vi "Get Rx Hardware Channel Data.vi"(8 "error in":errorcluster, 11 "custom device ref in":T1 format="%.0x") -> (0 "error out":errorcluster, 1 "Rx hardware channel data":T2[](array[typedef]) {"labels settings for RT"."Label Timestamp Channel Data Reference" format="%.0x"; "labels settings for RT"."Word Initial Raw Value" format="%032.0f"; "labels settings for RT"."Label Disable/Trigger Channel Reference" format="%.0x"; "labels settings for RT"."parameter driver data"."Tx parameter refs" format="%.0x"; "labels settings for RT"."parameter driver data"."Rx block data refs"."Data Reference" format="%.0x"; "labels settings for RT"."SDI" format="%02b"; "labels settings for RT"."label" format="%.0o"}, 2 "incoming channels":T1[](array[typedef]) format="%.0x", 3 "custom device ref out":T1 format="%.0x")   [LabVIEW 2020]
uses:
  <vilib>/NI VeriStand/Custom Device API/Custom Device API.lvlib
  Scripting/Ballard ARINC 429 Scripting.lvlib
  <vilib>/NI VeriStand/Custom Device API/Data Access Type.ctl
  <vilib>/NI VeriStand/Custom Device API/Custom Device Item Ref.ctl
  Label.ctl
  Encoding and Decoding/Encoding.ctl
  Encoding and Decoding/Encoding and Decoding.lvlib
  <vilib>/NI VeriStand/Custom Device API/Data Reference.ctl
  <vilib>/NI VeriStand/Custom Device API/Block Data Reference.ctl
  RT Parameters.ctl
  RT Label Settings.ctl
  RT Hardware Channel Settings.ctl
  Transfer Type.ctl
  Parameter Definition.ctl
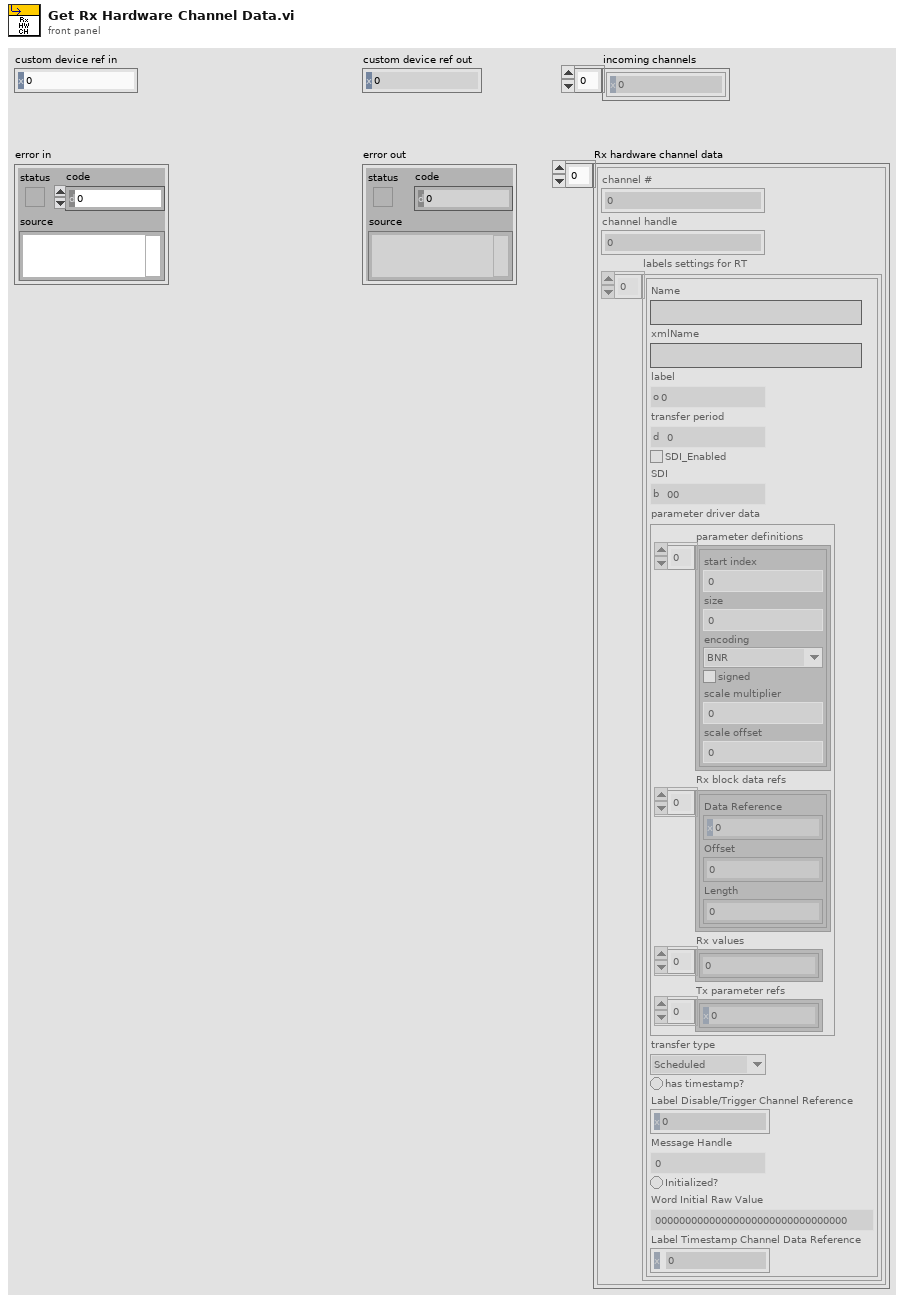
[diagram p1: front panel]
types:
  T1 = typedef "Custom Device API.lvlib/Custom Device Item Ref.ctl" = u64
  T2 = typedef "RT Hardware Channel Settings.ctl" = cluster{"channel #":u16, "channel handle":u64, "labels settings for RT":T3[]}
  T3 = typedef "RT Label Settings.ctl" = cluster{"Name":string, "xmlName":string, "label":T4, "transfer period":u32, "SDI_Enabled":bool, "SDI":u8, "parameter driver data":T5, "transfer type":T10, "has timestamp?":bool, "Label Disable/Trigger Channel Reference":T1, "Message Handle":u64, "Initialized?":bool, "Word Initial Raw Value":u32, "Label Timestamp Channel Data Reference":T9}
  T4 = typedef "Label.ctl" = u8
  T5 = typedef "RT Parameters.ctl" = cluster{"parameter definitions":T6[], "Rx block data refs":T8[], "Rx values":dbl[], "Tx parameter refs":T1[]}
  T6 = typedef "Parameter Definition.ctl" = cluster{"start index":i32, "size":i32, "encoding":T7, "signed":bool, "scale multiplier":dbl, "scale offset":dbl}
  T7 = typedef "Encoding and Decoding.lvlib/Encoding.ctl" = enum16{"BNR", "BCD", "Discrete"}
  T8 = typedef "Custom Device API.lvlib/Block Data Reference.ctl" = cluster{"Data Reference":T9, "Offset":u64, "Length":u64}
  T9 = typedef "Custom Device API.lvlib/Data Reference.ctl" = i32
  T10 = typedef "Transfer Type.ctl" = enum16{"Scheduled", "Acyclic", "Block", "Strobe"}
  T11 = typedef "Custom Device API.lvlib/Data Access Type.ctl" = enum16{"Read", "Write"}
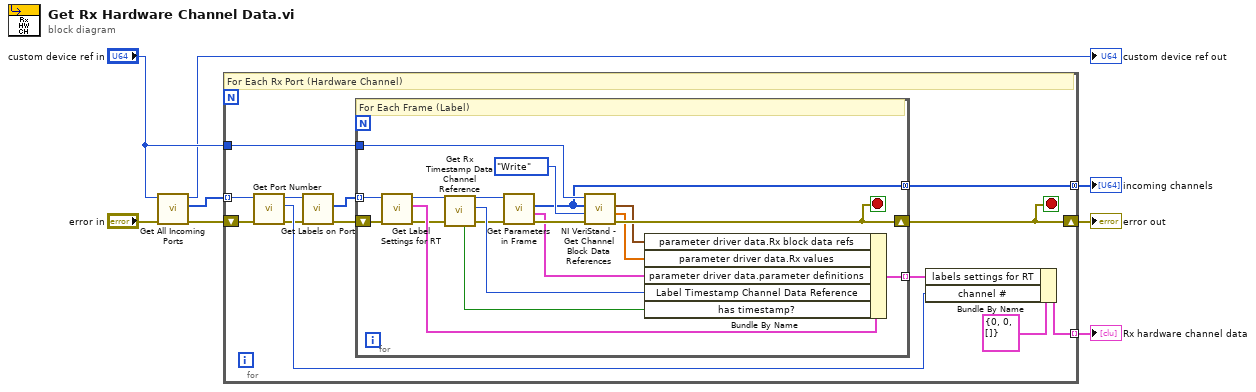
[diagram p0: block diagram]
diagram:
  n1 = call "Get All Incoming Ports.vi"("error in"="error in", "Ballard ARINC 429 ref"="custom device ref in") -> ("error out"=w5:errorcluster, "Port refs"=w4:T1[], "Ballard ARINC 429 ref out"=→"custom device ref out":T1)  [unwired: 7 in]
  n2 = for {
    tunnel: "custom device ref in" -> [w21]
    shift-right: [w20] -> w7
    shift-left: w5 -> [w15]
    tunnel: w4 -> [w16] mode=indexing
    tunnel: [w19] -> w6 mode=indexing
    tunnel: [w9] -> w1 mode=concatenating
    stop <- w20 stop-if-true
    # "For Each Rx Port (Hardware Channel)"
    n3 = call "Get Port Number.vi"("error in"=w15, "port ref in"=w16) -> ("error out"=w12:errorcluster, "port number"=w14:u16, "port ref out"=w13:T1)  [unwired: 6 in, 1 out]
    n4 = call "Get Labels on Port.vi"("error in"=w12, "port ref"=w13) -> ("error out"=w10:errorcluster, "label references"=w11:T1[])  [unwired: 6 in, 2 out]
    n5 = for {
      tunnel: w11 -> [w39] mode=indexing
      tunnel: w21 -> [w33]
      shift-right: [w29] -> w20
      shift-left: w10 -> [w38]
      tunnel: [w23] -> w18 mode=indexing
      tunnel: [w22] -> w9 mode=concatenating
      stop <- w29 stop-if-true
      # "For Each Frame (Label)"
      n6 = call "Get Label Settings for RT.vi"("error in"=w38, "label ref in"=w39) -> ("error out"=w34:errorcluster, "label settings for RT"=w36:T3, "label ref out"=w28:T1)  [unwired: 7 in]
      n7 = call "Get Rx Timestamp Data Channel Reference.vi"("error in"=w34, "frame ref in"=w28) -> ("error out"=w31:errorcluster, "timestamp channel data reference"=w32:T9, "frame ref out"=w30:T1, "timestamp channel found?"=w27:bool)  [unwired: 6 in]
      n8 = call "Get Parameters in Frame.vi"("error in"=w31, "frame ref in"=w30) -> ("error out"=w37:errorcluster, "parameter definitions"=w35:T6[], "parameter references"=w22:T1[])  [unwired: 6 in, 1 out]
      n9 = call <vilib>:"NI VeriStand - Get Channel Block Data References.vi"("error in (no error)"=w37, "Access"=Data_Access_Type."Write", "Channel Refs"=w22, "Device Ref in"=w33) -> ("error out"=w29:errorcluster, "Values Array"=w25:dbl[], "Block Data Refs"=w24:T8[])  [unwired: 4 in, 1 out]
      n10 = Bundle By Name(cluster=w36, "parameter driver data.Rx block data refs"=w24, "parameter driver data.Rx values"=w25, "parameter driver data.parameter definitions"=w35, "Label Timestamp Channel Data Reference"=w32, "has timestamp?"=w27) -> (w23:T3)
    }
    n11 = Bundle By Name(cluster=T2 {"channel #"=0, "channel handle"=0, "labels settings for RT"=[]} ("RT hardware channel"), "labels settings for RT"=w18, "channel #"=w14) -> (w19:T2)
  }
  "error out" <- w7
  "Rx hardware channel data" <- w6
  "incoming channels" <- w1
